vi "Module for APVSG.vi"(10 "Main controller mailbox":T2, 11 "THz module mailbox":T2) -> (2 "Ended":bool, 3 "Connected":bool)   [LabVIEW 2024, in "THz source modeule.lvlib"]
doc: "Module to set constant frequency or simple frequency sweep on RF (main) synthesizer and offset frequency on LO (folowing) synthesizer.\nKey typedefs: THz_Message for module, THz_Comands enum (Ignore, Initialize, Update, Set parameters, Disconnect, End), THz_Sweeep parameters\n***Note: This is old-fashoed module. Shall be replaced by newer.***\nComands and responses:\nInitialize: VDI config constants {Master{lower limit, upper limit, name, handle, description}, Follower{ lower limit, upper limit, name, handle, description } } (cluster of two clusters {numeric, numeric, string, numeric, string}) / handle log (string)\nUpdate: - / M_ID F_ID (string)\nSet parameters: Sweep parameters {Start, End, Sweep up time, Sweep down time, Intermediate, Reset trigger} (cluster{numeric, numeric, numeric, numeric, numeric, boolean}) / Sweep parameters (same cluster)\nDisconnect: - / master and follower name (string)\nEnd: - / Master and Follower handle (string)"
uses:
  THz source modeule.lvlib
  Messenger service/Data types/Mailbox address.ctl
  ctl/THz MW generator constants.ctl
  Messenger service/Data types/Module name.ctl
  ctl/THz sweep parameters.ctl
  ctl/THz Message for module.ctl
  ctl/THz commands enum.ctl
  <vilib>/ErrorRing/Error Ring.xnode
  <instrlib>/APVSG/APVSG20.lvlib
  Messenger service/MessengerLib.lvlib
panel:
  out "Constants":T1[](array[typedef])
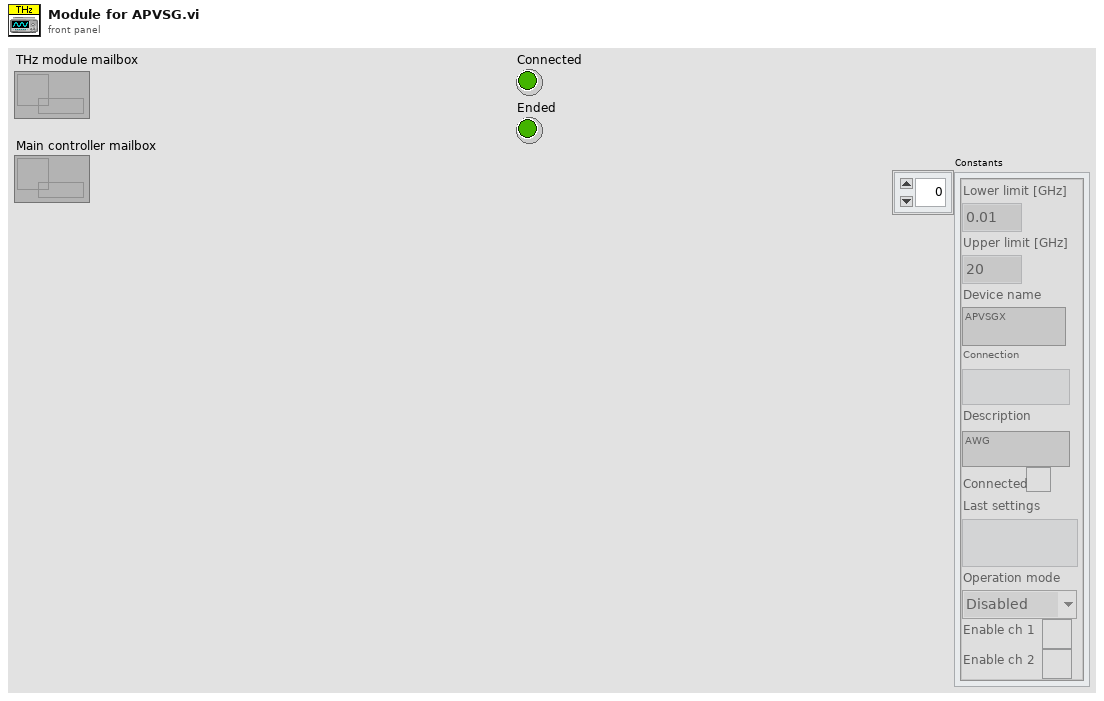
[diagram p1: front panel]
types:
  T1 = typedef "THz source modeule.lvlib/THz MW generator constants.ctl" = cluster{"Lower limit [GHz]":dbl, "Upper limit [GHz]":dbl, "Device name":string, "Connection":string, "Description":string, "Connected":bool, "Last settings":string, "Operation mode":enum16{"Disabled", "CW", "Arbitrary", "Sweep"}, "Enable ch 1":bool, "Enable ch 2":bool}
  T2 = typedef "MessengerLib.lvlib/Mailbox address.ctl" = refnum<queue>
  T3 = typedef "THz source modeule.lvlib/THz Message for module.ctl" = cluster{"Command":T4, "Data":variant}
  T4 = typedef "THz source modeule.lvlib/THz commands enum.ctl" = enum16{"Ignore", "Connect", "Update", "Set parameters", "Disconnect", "End"}
  T5 = typedef "THz source modeule.lvlib/THz sweep parameters.ctl" = cluster{"Start [GHz]":dbl, "End [GHz] ":dbl, "Sweep up\ntime [ms]":dbl, "Sweep down\ntime [ms]":dbl, "Intermidiate [MHz]":dbl, "Reset trigger":bool}
  T6 = typedef "Module name.ctl" = enum16{"Emty", "Magnet", "VTI", "Excitation", "Servo", "Acquisition", "Rotator", "Digitizer", "SMU2450", "Carousel", "Multimeter", "Tmp monitor", "Power monitor"}
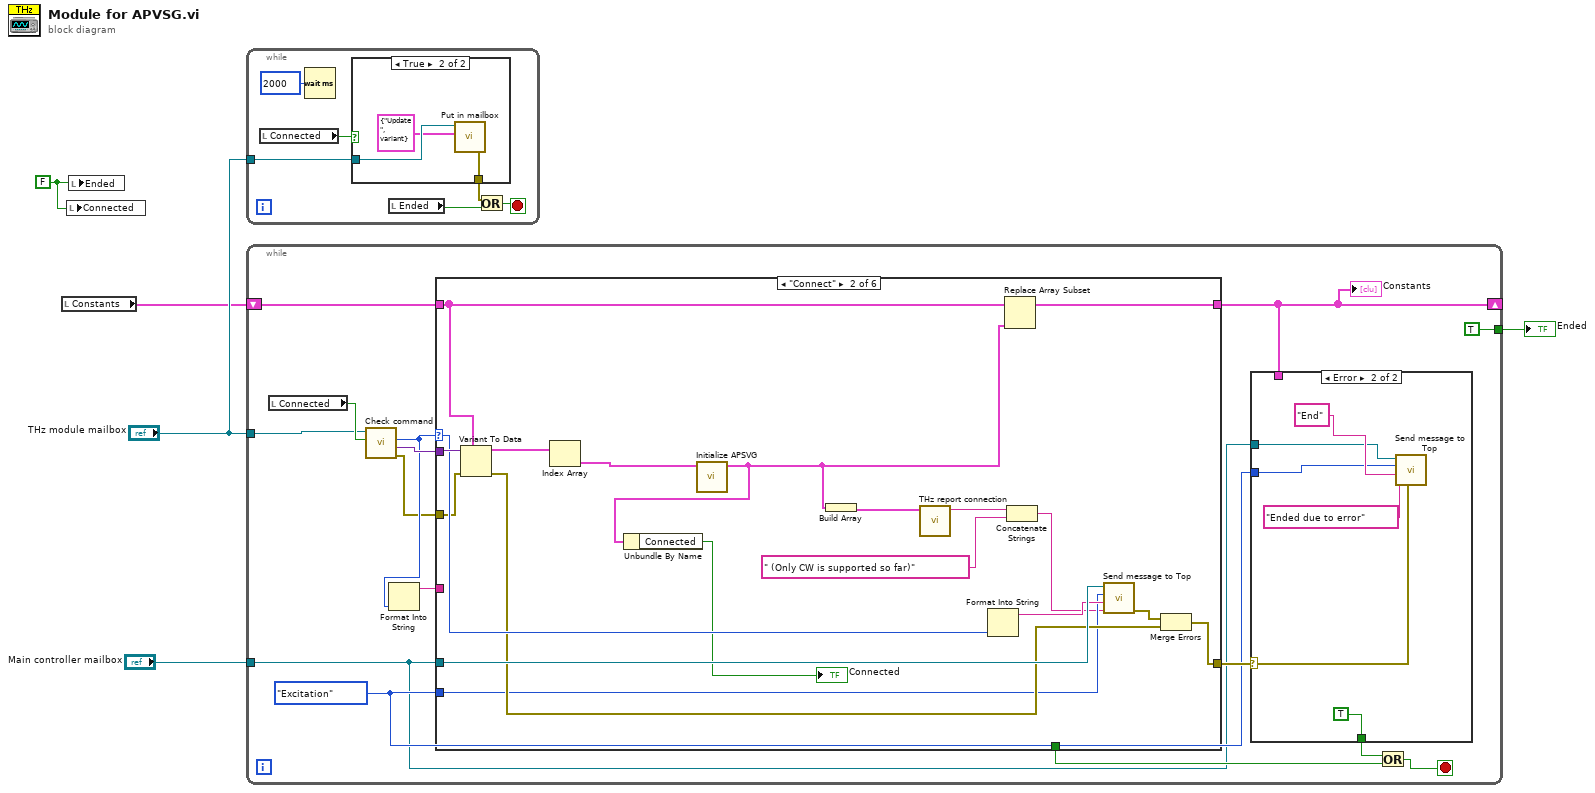
[diagram p0: block diagram]
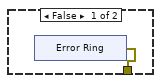
[diagram p2: hidden frame]
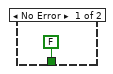
[diagram p3: hidden frame]
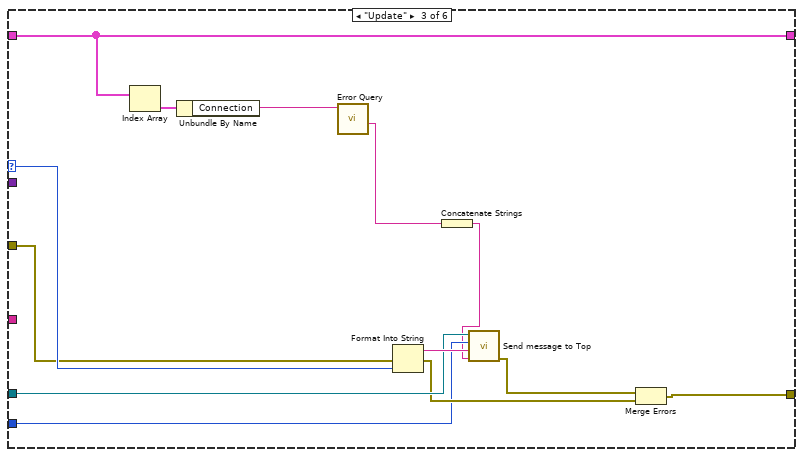
[diagram p5: hidden frame]
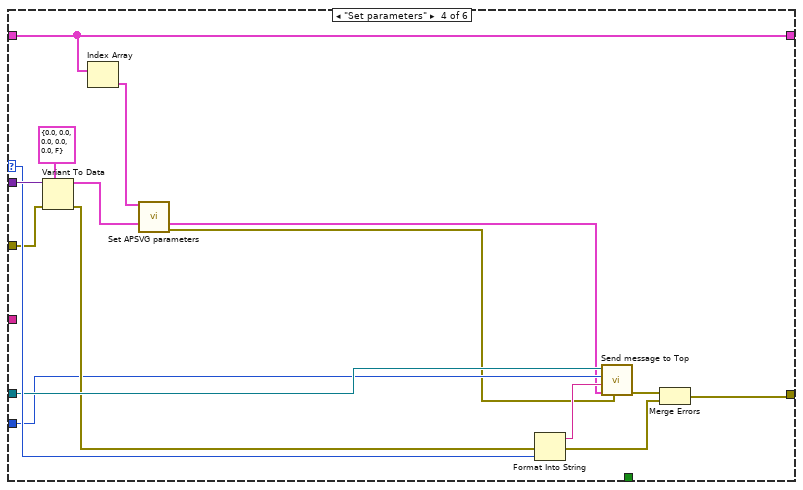
[diagram p6: hidden frame]
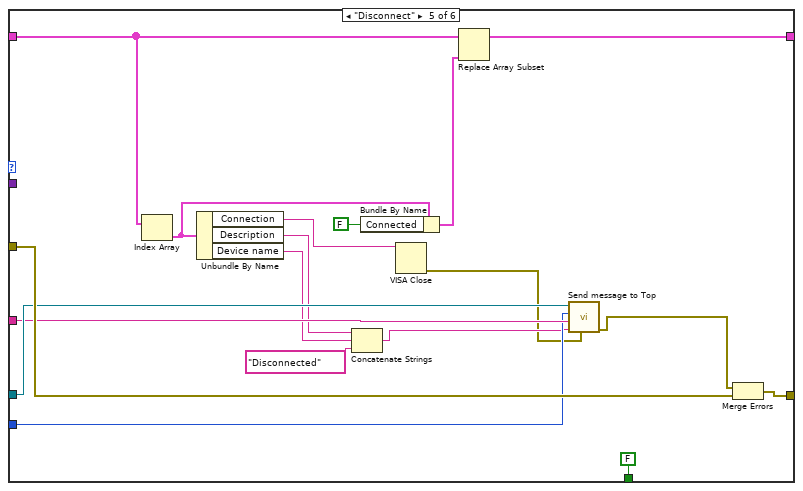
[diagram p7: hidden frame]
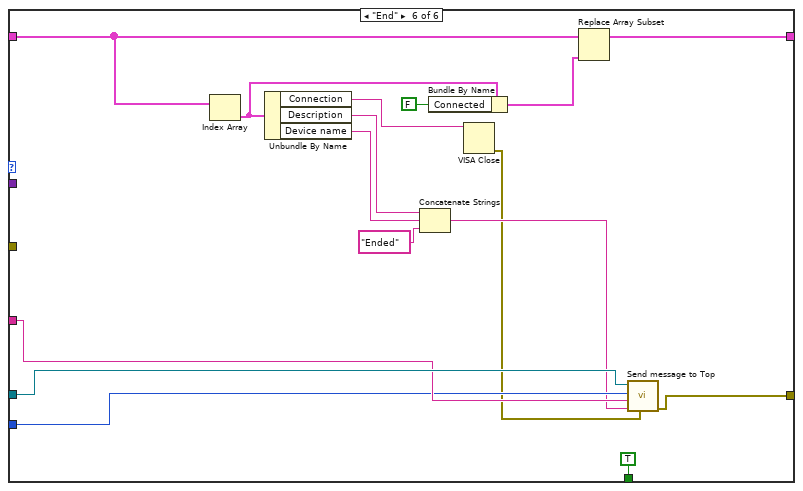
[diagram p8: hidden frame]
diagram:
  w1 = FALSE ("Initialized")
  n1 = local read "Constants"() -> (w3:T1[])
  n2 = local write "Connected"(w1) -> ()
  n3 = local write "Ended"(w1) -> ()
  n4 = while {
    tunnel: "THz module mailbox" -> [w9]
    stop <- w8 stop-if-true
    n5 = local read "Connected"() -> (w10:bool)
    n6 = Wait (ms)(milliseconds to wait=u32 2000) -> ()  [unwired: 1 out]
    n7 = case shown="True" w10 {
      tunnel: w9 -> [_ w16]
      tunnel: [w12 w14] -> w7
      frame False {
        n8 = xnode "Error Ring"() -> ("error out"=w12:errorcluster)
      }
      frame True {
        n9 = call "Put in mailbox.vi"("Message"=T3 {"Command"=enum."Update", "Data"=variant} ("Incoming msg"), "Queue in"=w16) -> ("error out"=w14:errorcluster)  [unwired: 7 in, 2 out]
      }
    }
    n10 = local read "Ended"() -> (w6:bool)
    n11 = Or(x=w7, y=w6) -> (x .or. y?=w8:bool)
  }
  n12 = while {
    shift-right: [w28] -> _
    shift-left: w3 -> [w31]
    tunnel: "THz module mailbox" -> [w20]
    tunnel: "Main controller mailbox" -> [w17]
    tunnel: [TRUE ("Initialized")] -> w2
    stop <- w26 stop-if-true
    w18 = Module_name."Excitation" ("Module")
    n13 = local read "Connected"() -> (w29:bool)
    n14 = call "Check command.vi"("Is connected"=w29, "Module mailbox"=w20) -> ("error out"=w19:errorcluster, "Command Data"=w30:variant, "Command"=w22:T4)  [unwired: 3 in]
    n15 = Format Into String(w22) -> (resulting string=w21:string)  [unwired: 3 in, 1 out]
    n16 = case shown="\"Connect\"" w22 {
      selector: w22 -> [_ w58 w71 w85 _ _]
      tunnel: [w40 w44 w63 w76 w93 w110] -> w28
      tunnel: w31 -> [w40 w45 w63 w76 w97 w111]
      tunnel: w30 -> [_ w59 _ w88 _ _]
      tunnel: [_ _ _ _ FALSE TRUE] -> w27
      tunnel: w17 -> [_ w57 w70 w84 w104 w122]
      tunnel: [w39 w55 w68 w81 w105 w121] -> w23
      tunnel: w19 -> [w39 w53 w67 w83 w106 _]
      tunnel: w18 -> [_ w51 w65 w78 w102 w119]
      tunnel: w21 -> [_ _ _ _ w103 w120]
      frame "Ignore", Default {
      }
      frame "Connect" {
        n17 = Variant To Data(error in=w53, type=w45, Variant=w59) -> (data=w50:T1[], error out=w52:errorcluster)
        n18 = Index Array(array=w50) -> (element=w49:T1)  [unwired: 1 in]
        n19 = call "Initialize APSVG.vi"("MW generator constants"=w49) -> ("MW generator constants out"=w43:T1)  [unwired: 5 in, 5 out]
        n20 = Unbundle By Name(w43) -> ("Connected"=→"Connected":bool)
        n21 = Build Array(w43) -> (w48:T1[])
        n22 = call "THz report connection.vi"("THz MW generator constants"=w48) -> ("string out"=w47:string)  [unwired: 10 in]
        n23 = Format Into String(w58) -> (resulting string=w56:string)  [unwired: 3 in, 1 out]
        n24 = Replace Array Subset(array=w45, new element=w43) -> (w44:T1[])  [unwired: 1 in]
        n25 = Concatenate Strings(w47, " (Only CW is supported so far)" ("string")) -> (w42:string)
        n26 = call "Send message to Top.vi"("Data"=w42, "Response"=w56, "Module"=w51, "Mailbox address in"=w57) -> ("Error out"=w54:errorcluster)  [unwired: 6 in, 1 out]
        n27 = Merge Errors(w54, w52) -> (w55:errorcluster)
      }
      frame "Update" {
        n28 = Index Array(array=w63) -> (element=w62:T1)  [unwired: 1 in]
        n29 = Unbundle By Name(w62) -> ("Connection"=w61:string)
        n30 = call <instrlib>:"Error Query.vi"("VISA resource in"=w61) -> ("Error Message"=w60:string)  [unwired: 7 in, 3 out]
        n31 = Format Into String(error in=w67, w71) -> (resulting string=w72:string, error out=w66:errorcluster)  [unwired: 2 in]
        n32 = Concatenate Strings(w60) -> (w64:string)
        n33 = call "Send message to Top.vi"("Data"=w64, "Response"=w72, "Module"=w65, "Mailbox address in"=w70) -> ("Error out"=w69:errorcluster)  [unwired: 6 in, 1 out]
        n34 = Merge Errors(w69, w66) -> (w68:errorcluster)
      }
      frame "Set parameters" {
        n35 = Variant To Data(error in=w83, type=T5 {"Start [GHz]"=0.0, "End [GHz] "=0.0, "Sweep up\ntime [ms]"=0.0, "Sweep down\ntime [ms]"=0.0, "Intermidiate [MHz]"=0.0, "Reset trigger"=FALSE} ("Sweep parameters"), Variant=w88) -> (data=w77:T5, error out=w82:errorcluster)
        n36 = Index Array(array=w76) -> (element=w75:T1)  [unwired: 1 in]
        n37 = call "Set APSVG parameters.vi"("Signal generator configuration"=w75, "Sweep parameters"=w77) -> ("Sweep parameters out"=w73:T5, "error out"=w74:errorcluster)  [unwired: 11 in, 1 out]
        n38 = Format Into String(error in=w82, w85) -> (resulting string=w86:string, error out=w80:errorcluster)  [unwired: 2 in]
        n39 = call "Send message to Top.vi"("Error in (no error)"=w74, "Data"=w73, "Response"=w86, "Module"=w78, "Mailbox address in"=w84) -> ("Error out"=w79:errorcluster)  [unwired: 5 in, 1 out]
        n40 = Merge Errors(w79, w80) -> (w81:errorcluster)
      }
      frame "Disconnect" {
        n41 = Index Array(array=w97) -> (element=w92:T1)  [unwired: 1 in]
        n42 = Unbundle By Name(w92) -> ("Connection"=w96:string, "Description"=w94:string, "Device name"=w95:string)
        n43 = Concatenate Strings(w94, w95, "Disconnected" ("string")) -> (w98:string)
        n44 = Bundle By Name(cluster=w92, "Connected"=FALSE) -> (w90:T1)
        n45 = VISA Close(VISA resource name=w96) -> (error out=w89:errorcluster)  [unwired: 1 in]
        n46 = Replace Array Subset(array=w97, new element=w90) -> (w93:T1[])  [unwired: 1 in]
        n47 = call "Send message to Top.vi"("Error in (no error)"=w89, "Data"=w98, "Response"=w103, "Module"=w102, "Mailbox address in"=w104) -> ("Error out"=w100:errorcluster)  [unwired: 5 in, 1 out]
        n48 = Merge Errors(w100, w106) -> (w105:errorcluster)
      }
      frame "End" {
        n49 = Index Array(array=w111) -> (element=w114:T1)  [unwired: 1 in]
        n50 = Unbundle By Name(w114) -> ("Connection"=w117:string, "Description"=w115:string, "Device name"=w116:string)
        n51 = Concatenate Strings(w115, w116, "Ended" ("string")) -> (w108:string)
        n52 = Bundle By Name(cluster=w114, "Connected"=FALSE) -> (w109:T1)
        n53 = VISA Close(VISA resource name=w117) -> (error out=w107:errorcluster)  [unwired: 1 in]
        n54 = Replace Array Subset(array=w111, new element=w109) -> (w110:T1[])  [unwired: 1 in]
        n55 = call "Send message to Top.vi"("Error in (no error)"=w107, "Data"=w108, "Response"=w120, "Module"=w119, "Mailbox address in"=w122) -> ("Error out"=w121:errorcluster)  [unwired: 5 in, 1 out]
      }
    }
    "Constants" <- w28
    n56 = case shown="Error" w23 {
      selector: w23 -> [_ w33]
      tunnel: w28 -> [_ _]
      tunnel: [FALSE TRUE] -> w25
      tunnel: w18 -> [_ w36]
      tunnel: w17 -> [_ w35]
      frame No Error {
      }
      frame Error {
        n57 = call "Send message to Top.vi"("Error in (no error)"=w33, "Data"="Ended due to error", "Response"="End", "Module"=w36, "Mailbox address in"=w35) -> ()  [unwired: 5 in, 2 out]
      }
    }
    n58 = Or(x=w25, y=w27) -> (x .or. y?=w26:bool)
  }
  "Ended" <- w2
